vi "solstis_change_wavelength.vi"(8 "error in (no error)":errorcluster, 10 "Setpoint(nm)":dbl=770.808543 format="%#_13g", 11 "connection ID":refnum<k5>) -> (0 "error out":errorcluster, 1 "Change wavelength outputs":string[](array[string]), 2 "data out":string="{\"message\":{\"transmission_id\":[3],\"op\":\"parse_fail\",\"parameters\":{\"protocol_error\":[1],\"JSON_parse_error\":\"\"}}}", 3 "connection ID out":refnum<k5>)   [LabVIEW 2017]
panel:
  out "F-format string":string
  in  "Tx":i32=2
  in  "operation":string="\"set_wave_m\""
  # "parameter values"
  # "to access solstis main console open web browser and type its IP address.\nusername: main  password: main\nnetwork settings under configure, make sure remote interface IP address matches\n lab PC IP address\n\nLab PC needs IPV4 static IP address 192.168.1.xxx, xxx is 3 numbers\nsubnet mask 255.255.255.0\ndefault gateway 192.168.1.1\nIn NI MAX set up a network device with the IP address of the Solstis and \nthe port listed in the solstis network settings for remote interface.\n\nIn solstis network settings give wavemeter same address as PC but a different port, \nmatching what is in the wavemeter server software."
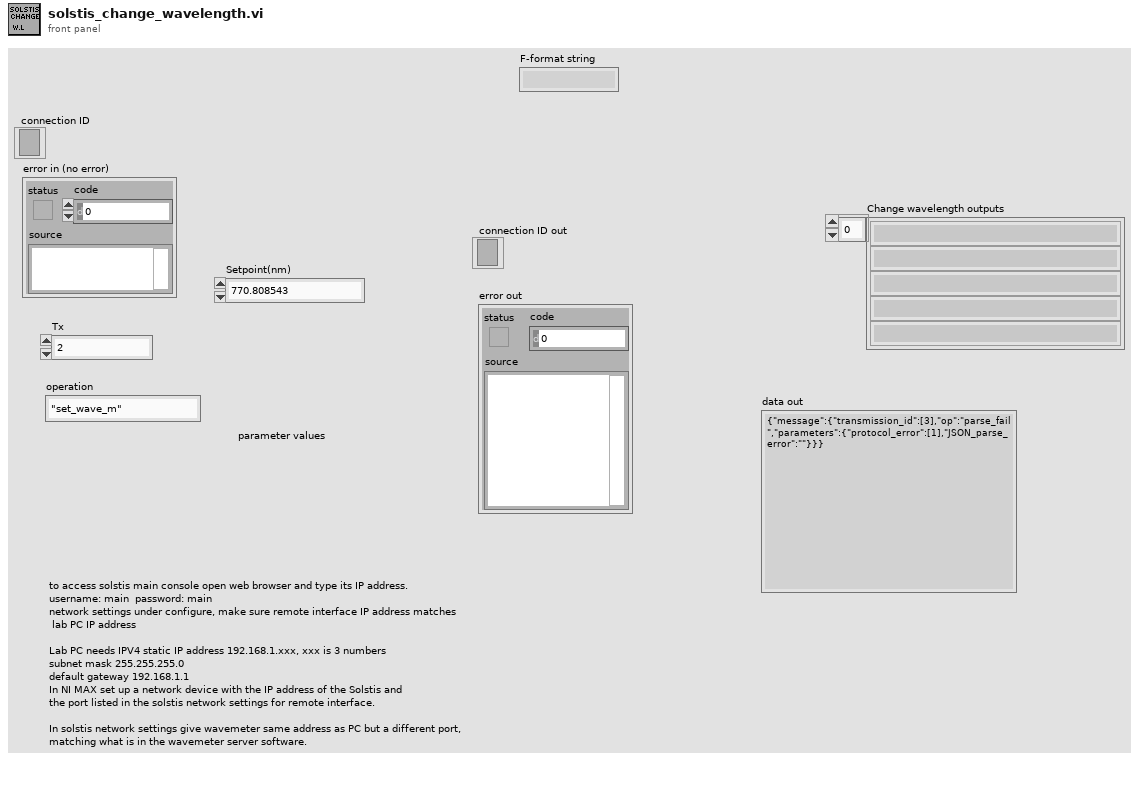
[diagram p1: front panel]
types:
  T1 = enum16{"Standard", "Buffered", "CRLF", "Immediate"}
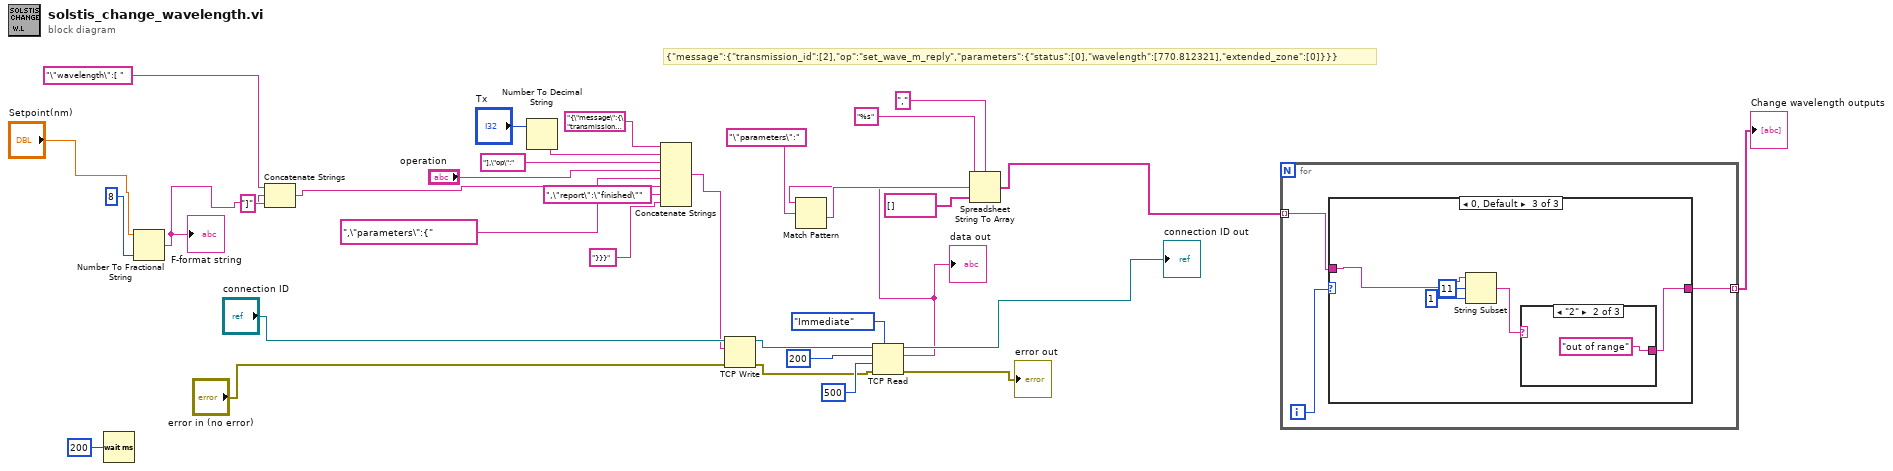
[diagram p0: block diagram]
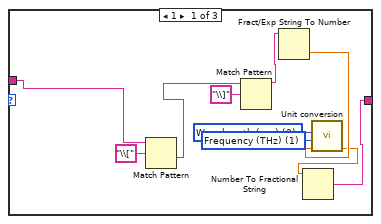
[diagram p2: hidden frame]
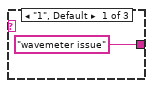
[diagram p4: hidden frame]
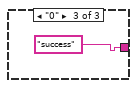
[diagram p5: hidden frame]
diagram:
  # "{\"message\":{\"transmission_id\":[2],\"op\":\"set_wave_m_reply\",\"parameters\":{\"status\":[0],\"wavelength\":[770.812321],\"extended_zone\":[0]}}}"
  n1 = Wait (ms)(milliseconds to wait=u32 200) -> ()  [unwired: 1 out]
  n2 = Number To Fractional String(number="Setpoint(nm)", precision (6)=i16 8) -> (F-format string=w13:string)  [unwired: 2 out]
  "F-format string" <- w13
  n3 = Concatenate Strings("\"wavelength\":[ ", w13, "]" ("string")) -> (w18:string)
  n4 = Number To Decimal String(number="Tx") -> (decimal integer string=w23:string)  [unwired: 1 out]
  n5 = Concatenate Strings("{\"message\":{\"transmission_id\":[" ("string"), w23, "],\"op\":" ("string"), "operation", ",\"parameters\":{" ("string"), w18, ",\"report\":\"finished\"" ("string"), "}}}" ("string")) -> (w10:string)
  n6 = TCP Write(connection ID="connection ID", data in=w10, error in (no error)="error in (no error)") -> (connection ID out=w32:refnum<k5>, error out=w1:errorcluster)  [unwired: 2 out]
  n7 = TCP Read(connection ID=w32, bytes to read=200, error in (no error)=w1, 7:T1."Immediate" ("mode (standard)"), 9:500 ("timeout ms (25000)")) -> (connection ID out=→"connection ID out":refnum<k5>, data out=w4:string, error out=→"error out":errorcluster)
  "data out" <- w4
  n8 = Match Pattern(string=w4, regular expression="\"parameters\":") -> (after substring=w8:string)  [unwired: 4 out]
  n9 = Spreadsheet String To Array(delimiter (Tab)=",", format string="%s", spreadsheet string=w8, array type (2D Dbl)=string[] []) -> (array=w3:string[])
  n10 = for {
    tunnel: w3 -> [w35] mode=indexing
    tunnel: [w34] -> w2 mode=indexing
    i -> [w36]
    n11 = case shown="0, Default" w36 {
      tunnel: w35 -> [w45 w47 w52]
      tunnel: [w37 w47 w48] -> w34
      frame 1 {
        w39 = u16 1 items=["Wavenumber (cm-1)", "Frequency (THz)", "Wavelength (nm)"] ("Ending Units")
        w41 = u16 2 items=["Wavenumber (cm-1)", "Frequency (THz)", "Wavelength (nm)"] ("Starting Units")
        n12 = Match Pattern(string=w45, regular expression="\\[") -> (after substring=w43:string)  [unwired: 4 out]
        n13 = Match Pattern(string=w43, regular expression="\\]") -> (before substring=w42:string)  [unwired: 4 out]
        n14 = Fract/Exp String To Number(string=w42) -> (number=w40:dbl)  [unwired: 4 out]
        n15 = call "Unit conversion.vi"("Value to convert"=w40, "Ending Units"=w39, "Starting Units"=w41) -> ("Output"=w38:dbl)  [unwired: 8 out]
        n16 = Number To Fractional String(number=w38) -> (F-format string=w37:string)  [unwired: 3 out]
      }
      frame 2 {
      }
      frame 0, Default {
        n17 = String Subset(string=w52, offset (0)=11, length (rest)=1 ("length (rest)")) -> (substring=w49:string)
        n18 = case shown="\"2\"" w49 {
          tunnel: ["wavemeter issue" "out of range" "success"] -> w48
          frame "1", Default {
          }
          frame "2" {
          }
          frame "0" {
          }
        }
      }
    }
  }
  "Change wavelength outputs" <- w2
